vi "Get_Router_Data.vi"() -> ()   [LabVIEW 2015]
panel:
  out "body 2":string
  out "body":string
  out "Total Bundle Consumption":string
  out "Current Session Consumption":string
  out "Download Speed":string
  out "Upload Speed":string
  out "Router Up time":string
  out "Number of connected users":i32=7
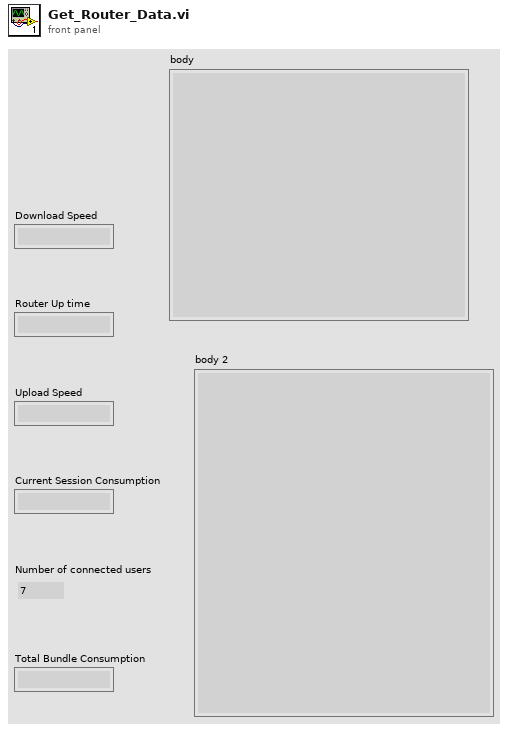
[diagram p1: front panel]
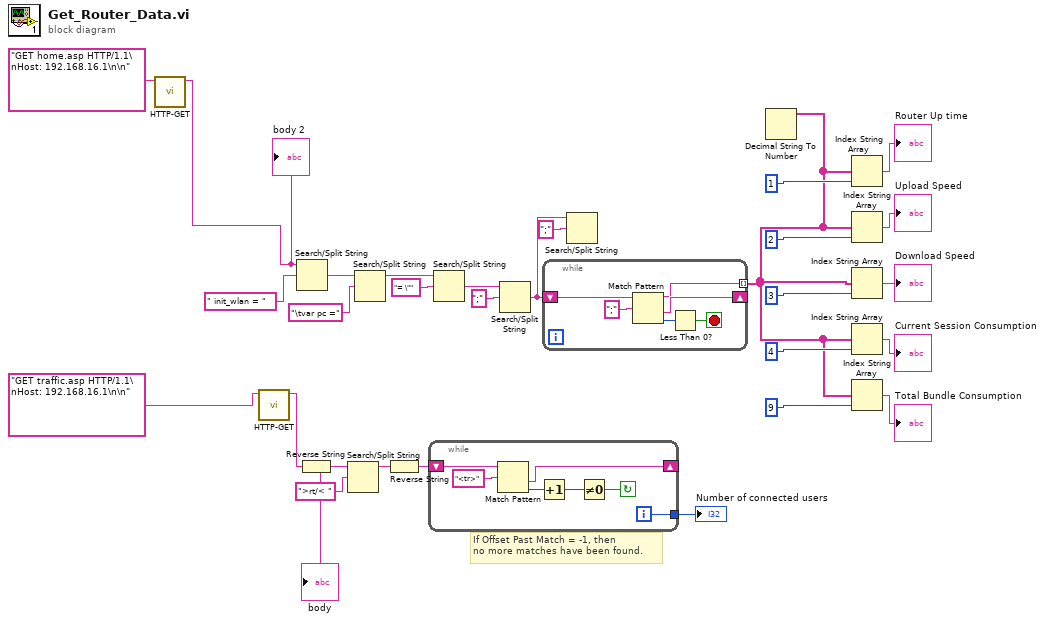
[diagram p0: block diagram]
diagram:
  # "If Offset Past Match = -1, then\nno more matches have been found."
  n1 = call "HTTP-GET.vi"("Command"="GET home.asp HTTP/1.1\nHost: 192.168.16.1\n\n") -> ("String"=w4:string)  [unwired: 10 in]
  "body 2" <- w4
  n2 = call "HTTP-GET.vi"("Command"="GET traffic.asp HTTP/1.1\nHost: 192.168.16.1\n\n") -> ("String"=w2:string)  [unwired: 10 in]
  "body" <- w2
  n3 = Search/Split String(string=w4, search string/char (-)=" init_wlan = ") -> (match + rest of string=w28:string)  [unwired: 1 in, 2 out]
  n4 = Reverse String(1:w2) -> (0:w20:string)
  n5 = Search/Split String(string=w20, search string/char (-)=">rt/< ") -> (substring before match=w18:string)  [unwired: 1 in, 2 out]
  n6 = Search/Split String(string=w28, search string/char (-)="\tvar pc =") -> (substring before match=w26:string)  [unwired: 1 in, 2 out]
  n7 = Reverse String(1:w18) -> (0:w16:string)
  n8 = while {
    tunnel: [w30] -> w17
    shift-left: w16 -> [w36]
    shift-right: [w34] -> _
    i -> [w30]
    stop <- w31 continue-if-true
    n9 = Match Pattern(string=w36, regular expression="<tr>") -> (after substring=w34:string, offset past match=w33:i32)  [unwired: 1 in, 2 out]
    n10 = Increment(x=w33) -> (x+1=w32:i32)
    n11 = Not Equal To 0?(x=w32) -> (x != 0?=w31:bool)
  }
  "Number of connected users" <- w17
  n12 = Search/Split String(string=w26, search string/char (-)="= \"") -> (match + rest of string=w24:string)  [unwired: 1 in, 2 out]
  n13 = Search/Split String(string=w24, search string/char (-)=";") -> (match + rest of string=w21:string)  [unwired: 1 in, 2 out]
  n14 = while {
    tunnel: [w39] -> w5 mode=indexing
    shift-right: [w40] -> _
    shift-left: w21 -> [w42]
    stop <- w37 stop-if-true
    n15 = Match Pattern(string=w42, regular expression=";") -> (before substring=w39:string, after substring=w40:string, offset past match=w38:i32)  [unwired: 2 out]
    n16 = Less Than 0?(x=w38) -> (x < 0?=w37:bool)
  }
  n17 = Search/Split String(string=w21, search string/char (-)=";") -> ()  [unwired: 1 in, 3 out]
  n18 = Decimal String To Number(string=w5) -> ()  [unwired: 4 out]
  n19 = Index String Array(1:1 ("index"), 2:w5) -> (0:→"Router Up time":string)  [unwired: 1 in]
  n20 = Index String Array(1:2 ("index"), 2:w5) -> (0:→"Upload Speed":string)  [unwired: 1 in]
  n21 = Index String Array(1:3 ("index"), 2:w5) -> (0:→"Download Speed":string)  [unwired: 1 in]
  n22 = Index String Array(1:4 ("index"), 2:w5) -> (0:→"Current Session Consumption":string)  [unwired: 1 in]
  n23 = Index String Array(1:9 ("index"), 2:w5) -> (0:→"Total Bundle Consumption":string)  [unwired: 1 in]
